vi "CDMA_RxTrchDecoder.vi"(8 "error in (no error)":errorcluster caption="错误输入（无错误）", 9 "rx_coder_type":dbl, 10 "dpchBit":dbl[](array[numeric]), 11 "Path In":path) -> (0 "error out":errorcluster caption="错误输出", 2 "ch_decode_data":dbl[](array[numeric]), 3 "Path Out":path)   [LabVIEW 2015]
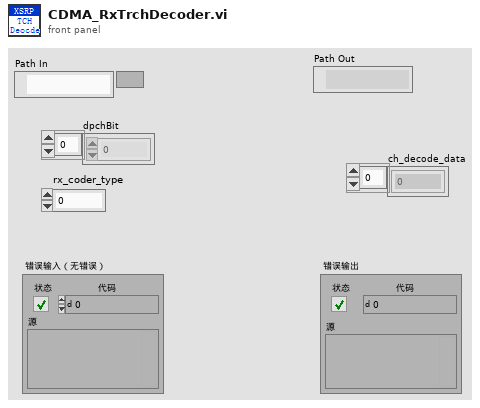
[diagram p1: front panel]
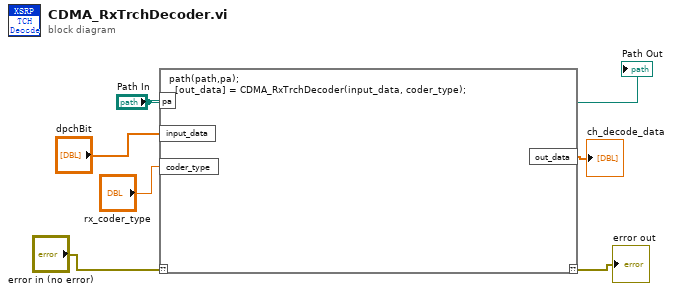
[diagram p0: block diagram]
diagram:
  n1 = script code="path(path,pa);\n  [out_data] = CDMA_RxTrchDecoder(input_data, coder_type);"("??"="error in (no error)", "pa"="Path In", "input_data"="dpchBit", "coder_type"="rx_coder_type") -> ("??"=→"error out":errorcluster, "out_data"=→"ch_decode_data":dbl[])
  "Path Out" <- "Path In"
